vi "ManualMajorityAdderTest.vi"() -> ()   [LabVIEW 2012]
uses:
  <vilib>/Utility/NIReport.llb/NI_report.lvclass
  <vilib>/Utility/NIReport.llb/HTML/NI_HTML.lvclass
  Sum_Abrilader/L0_Sum_Adder Folder/C/Program Files/National Instruments/LabVIEW 2012/instr.lib/Agilent 81150/Agilent 81150.lvlib
panel:
  in  "index":i8(slide)=4 min=0 max=4 step=1
  in  "stop":bool
  in  "Voltages":dbl[](array[numeric])=[0.05, 0.1, 0.2, 0.5, 0.8]
  in  "Enable 6":bool=TRUE
  in  "Enable 4":bool=TRUE
  in  "Enable 5":bool=TRUE
  in  "Enable 2":bool=TRUE
  in  "Enable 3":bool=TRUE
  in  "Enable 0":bool=TRUE
  in  "Enable 1":bool=TRUE
  in  "threshold":i32[][](array[numeric])=[[600, 600, 600, 600, 600, 600, 600], [600, 600, 600, 600, 600, 600, 600], [600, 600, 600, 600, 600, 600, 600], [600, 600, 600, 600, 600, 600, 600], [600, 600, 600, 600, 600, 600, 600]]
  out "error out":errorcluster
  in  "Instrument VISA in":T1={"AWG VISA"="AgilentGenerator1", "Oscilloscope  VISA "="AgilentOsciloscope", "Integration Board IP"="172.16.17.47", "connection ID"=refnum, "report out"=refnum, "report file path"=path "C:/Documents and Settings/CTA_LAB01/Desktop/L0_Asic/L0 Asic Test Data"}
  in  "error in":errorcluster
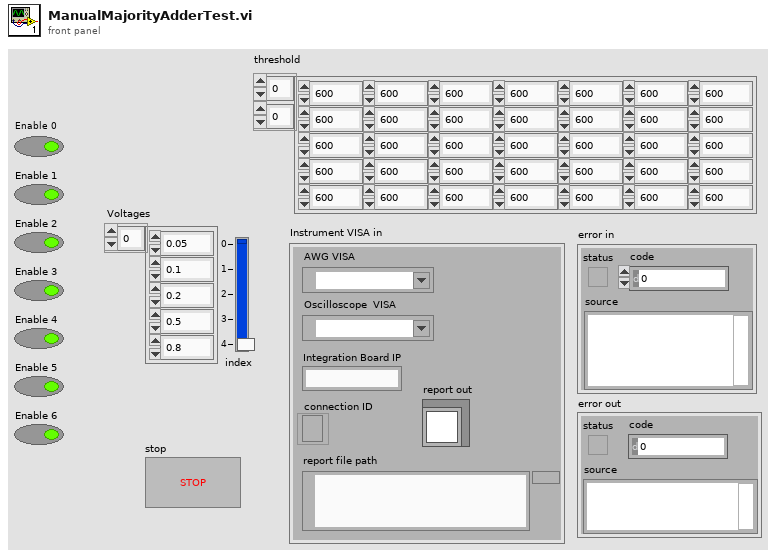
[diagram p1: front panel]
types:
  T1 = cluster{"AWG VISA":refnum<visa-resource-name>, "Oscilloscope  VISA ":refnum<visa-resource-name>, "Integration Board IP":string, "connection ID":refnum<k5>, "report out":refnum<class "NI_report.lvclass">, "report file path":path}
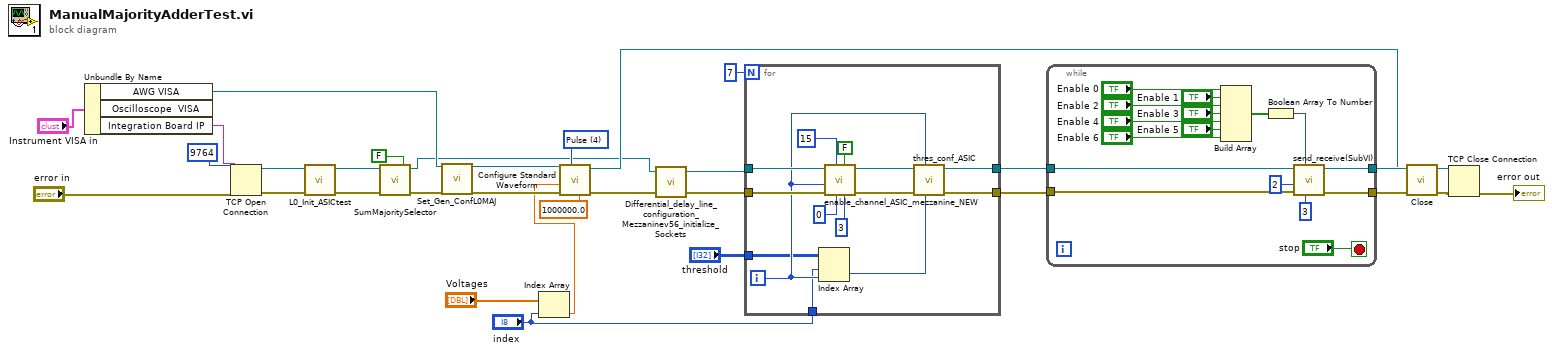
[diagram p0: block diagram]
diagram:
  w10 = u16 4 items=["Sine", "Square", "Ramp Up", "Ramp Down", "Pulse", "Noise", "DC"] ("Waveform (0: Sine)")
  n1 = Unbundle By Name("Instrument VISA in") -> ("AWG VISA"=w19:refnum<visa-resource-name>, "Integration Board IP"=w29:string)  [unwired: 1 out]
  n2 = TCP Open Connection(address=w29, remote port or service name=9764, error in (no error)="error in") -> (connection ID=w24:refnum<k5>, error out=w25:errorcluster)  [unwired: 2 in]
  n3 = call "L0_Init_ASICtest.vi"("error in"=w25, "connection ID in"=w24) -> ("error out"=w26:errorcluster, "connection ID out"=w23:refnum<k5>)  [unwired: 8 in]
  n4 = call "SumMajoritySelector.vi"("On Sum\nOff Majority"=FALSE ("On Sum\nOff Majority"), "error in (no error)"=w26, "connection ID"=w23) -> ("error out"=w20:errorcluster, "connection ID out"=w2:refnum<k5>)  [unwired: 5 in]
  n5 = call "Set_Gen_ConfL0MAJ.vi"("AWG VISA"=w19, "error in (no error)"=w20) -> ("VISA resource name out"=w16:refnum<visa-resource-name>, "error out"=w18:errorcluster)  [unwired: 10 in, 6 out]
  n6 = Index Array(array="Voltages", index="index") -> (element=w7:dbl)
  n7 = call <instrlib>:"Configure Standard Waveform.vi"("Frequency (1000.0 Hz)"=1000000.0, "Waveform (0: Sine)"=w10, "error in (no error)"=w18, "Amplitude (1.0 Vpp)"=w7, "VISA resource name"=w16) -> ("error out"=w4:errorcluster, "VISA resource name out"=w13:refnum<visa-resource-name>)  [unwired: 5 in]
  n8 = call "Differential_delay_line_configuration_Mezzaninev56_initialize_Sockets.vi"("connection ID"=w2, "error in (no error)"=w4) -> ("connection ID out"=w1:refnum<k5>, "error out 2"=w3:errorcluster)  [unwired: 6 in]
  n9 = for {
    N: 7 -> [_]
    tunnel: [w45] -> w6
    tunnel: w3 -> [w44]
    tunnel: w1 -> [w42]
    tunnel: [w40] -> w5
    tunnel: "threshold" -> [w34]
    tunnel: "index" -> [w32]
    i -> [w35]
    n10 = Index Array(array=w34, index (row)=w32, index (col)=w35) -> (element=w33:i32)
    n11 = call "enable_channel_ASIC_mezzanine_NEW.vi"("Clip_sel_b"=u32 3, "maj/sum"=FALSE, "Ib_clipVb"=u32 0, "Att gain"=u32 15, "error in"=w44, "Channel"=w35, "connection ID"=w42) -> ("error out"=w43:errorcluster, "connection ID out"=w41:refnum<k5>)  [unwired: 2 in, 1 out]
    n12 = call "thres_conf_ASIC.vi"("threshold"=w33, "Ring"=w35, "error out 3"=w43, "connection ID"=w41) -> ("error out 2"=w45:errorcluster, "connection ID out"=w40:refnum<k5>)  [unwired: 4 in, 2 out]
  }
  n13 = while {
    tunnel: [w61] -> w21
    tunnel: [w60] -> w15
    tunnel: w6 -> [w59]
    tunnel: w5 -> [w46]
    stop <- "stop" stop-if-true
    n14 = Build Array("Enable 0", "Enable 1", "Enable 2", "Enable 3", "Enable 4", "Enable 5", "Enable 6") -> (w57:bool[])
    n15 = Boolean Array To Number(Boolean array=w57) -> (number=w49:u32)
    n16 = call "send_receive(SubVI).vi"("Action"=3, "Data"=w49, "error in"=w59, "Address"=2, "connection ID"=w46) -> ("error out"=w60:errorcluster, "connection ID out"=w61:refnum<k5>)  [unwired: 2 in, 3 out]
  }
  n17 = call <instrlib>:"Close.vi"("error in (no error)"=w15, "VISA resource name"=w13) -> ("error out"=w14:errorcluster)  [unwired: 9 in]
  n18 = TCP Close Connection(connection ID=w21, error in (no error)=w14) -> (error out=→"error out":errorcluster)  [unwired: 1 in, 1 out]
